vi "Wrist Encoder Position to XZ Offset.vi"(9 "Wrist Offset (Inches)":dbl, 10 "Wrist Enc Pos":dbl) -> (0 "Wrist Z":dbl, 3 "Wrist X":dbl)   [LabVIEW 2023]
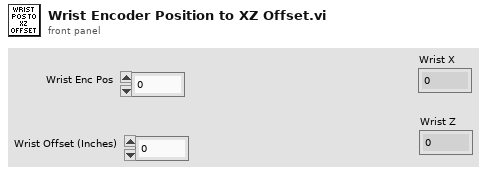
[diagram p1: front panel]
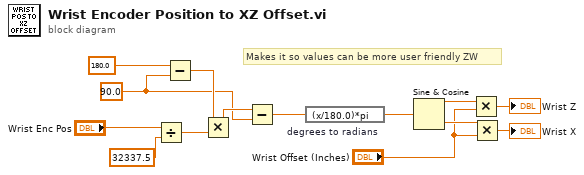
[diagram p0: block diagram]
diagram:
  w1 = 90.0 ("y")
  # "Makes it so values can be more user friendly ZW"
  n1 = Divide(x="Wrist Enc Pos", y=32337.5) -> (x/y=w7:dbl)
  n2 = Subtract(x=180.0, y=w1) -> (x-y=w6:dbl)
  n3 = Multiply(x=w6, y=w7) -> (x*y=w2:dbl)
  n4 = Subtract(x=w2, y=w1) -> (x-y=w4:dbl)
  n5 = expression code="(x/180.0)*pi" "degrees to radians"(w4) -> (w14:dbl)
  n6 = Sine & Cosine(0:w14) -> (1:w10:dbl, 2:w13:dbl)
  n7 = Multiply(x=w10, y="Wrist Offset (Inches)") -> (x*y=→"Wrist Z":dbl)
  n8 = Multiply(x=w13, y="Wrist Offset (Inches)") -> (x*y=→"Wrist X":dbl)
